vi "Select Active Channels.vi"(8 "error in (no error)":errorcluster, 9 "Impedance(s)":T1[](array[typedef]), 10 "Active Channel(s)":T2[](array[typedef]), 11 "MSOX6004 in":refnum<class "MSOX6004.lvclass">) -> (0 "error out":errorcluster, 3 "MSOX6004 out":refnum<class "MSOX6004.lvclass">)   [LabVIEW 2018, in "MSOX6004.lvlib" / "MSOX6004.lvclass"]
doc: "This Override method is used to set active channels for the Oscope. Use the 'Active Channel(s)' control to select channel(s)."
uses:
  MSOX6004.lvclass
  PPLs/Oscilloscope/Parent/Oscilloscope.lvlibp/Custom Controls/Analog Channels.ctl
  PPLs/Oscilloscope/Parent/Oscilloscope.lvlibp/Accessors/Channel Impedance.ctl
  MSOX6004.lvclass/MSOX6004.ctl
  <instrlib>/Keysight InfiniiVision/Keysight InfiniiVision.lvlib
  PPLs/Oscilloscope/Parent/Oscilloscope.lvlibp
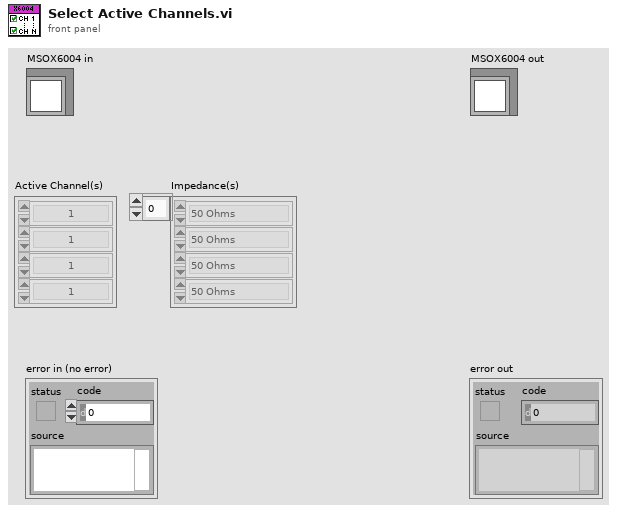
[diagram p1: front panel]
types:
  T1 = typedef "Oscilloscope.lvlibp/Channel Impedance.ctl" = enum16{"50 Ohms", "1 MOhms"}
  T2 = typedef "Oscilloscope.lvlibp/Analog Channels.ctl" = enum16{"1", "2", "3", "4", "5", "6", "7", "8", "9", "10", "11", "12", "13", "14", "15", "16"}
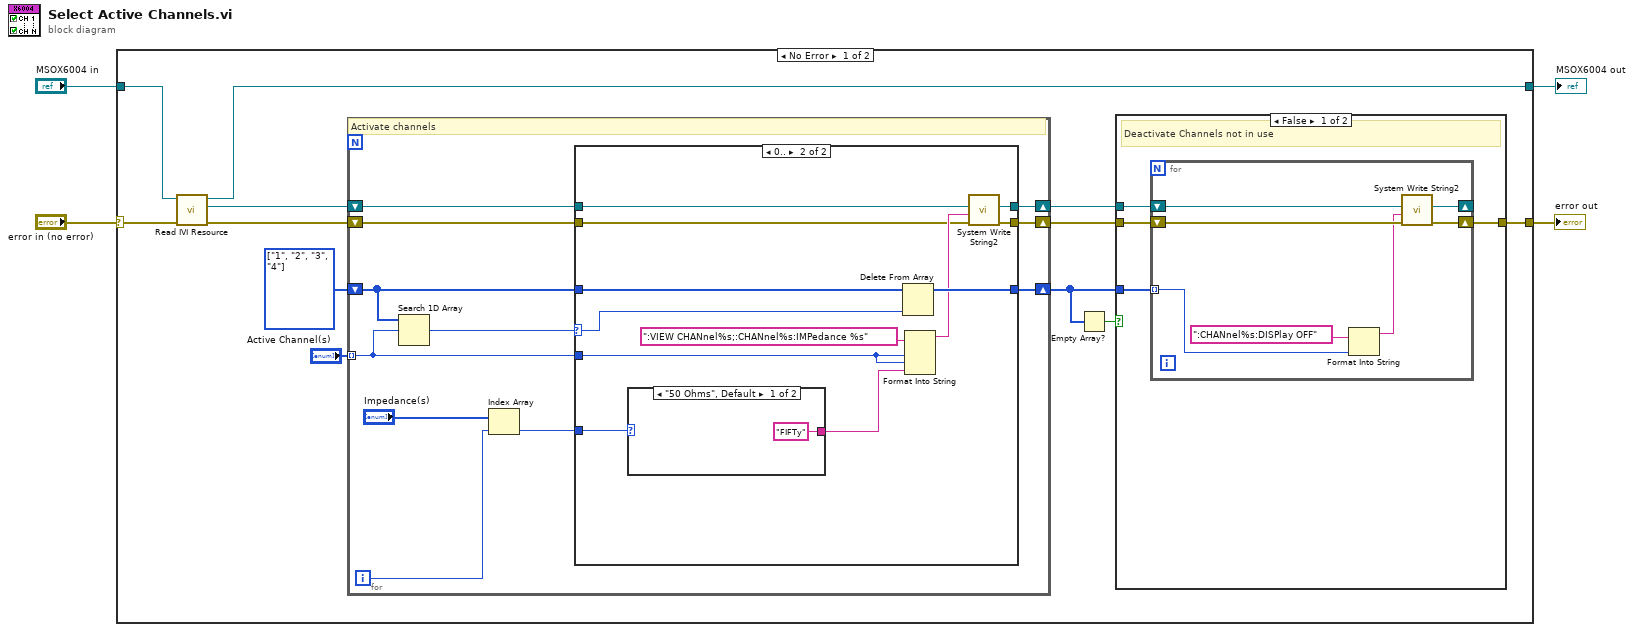
[diagram p0: block diagram]
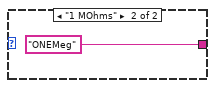
[diagram p4: hidden frame]
diagram:
  n1 = case shown="No Error" "error in (no error)" {
    selector: "error in (no error)" -> [w16 w57]
    tunnel: [w14 w58] -> w3
    tunnel: "MSOX6004 in" -> [w15 w58]
    tunnel: [w6 w57] -> w1
    frame No Error {
      w10 = T2[] [enum."1", enum."2", enum."3", enum."4"] items=["1", "2", "3", "4", "5", "6", "7", "8", "9", "10", "11", "12", "13", "14", "15", "16"] ("Active Channel(s)")
      n2 = call "Read IVI Resource.vi"("error in (no error)"=w16, "MSOX6004 in"=w15) -> ("error out"=w12:errorcluster, "IVI Resource"=w11:refnum<k15>, "MSOX6004 out"=w14:refnum<class "MSOX6004.lvclass">)  [unwired: 7 in]
      n3 = for {
        tunnel: "Active Channel(s)" -> [w38] mode=indexing
        shift-right: [w39] -> w7
        shift-left: w12 -> [w34]
        shift-right: [w35] -> w5
        shift-left: w10 -> [w36]
        shift-right: [w33] -> w8
        shift-left: w11 -> [w37]
        i -> [w29]
        # "Activate channels"
        n4 = Search 1D Array(1D array=w36, element=w38) -> (index of element=w31:i32)  [unwired: 1 in]
        n5 = Index Array(array="Impedance(s)", index=w29) -> (element=w30:T1)
        n6 = case shown="0.." w31 {
          selector: w31 -> [_ w50]
          tunnel: [w41 w54] -> w39
          tunnel: w38 -> [_ w44]
          tunnel: w37 -> [w42 w52]
          tunnel: w36 -> [w40 w51]
          tunnel: [w40 w49] -> w35
          tunnel: w34 -> [w41 w47]
          tunnel: [w42 w46] -> w33
          tunnel: w30 -> [_ w45]
          frame -1, Default {
          }
          frame 0.. {
            n7 = case shown="\"50 Ohms\", Default" w45 {
              tunnel: ["FIFTy" "ONEMeg"] -> w43
              frame "50 Ohms", Default {
              }
              frame "1 MOhms" {
              }
            }
            n8 = Delete From Array(array=w51, index=w50) -> (array with subset deleted=w49:T2[])  [unwired: 1 in, 1 out]
            n9 = Format Into String(format string=":VIEW CHANnel%s;:CHANnel%s:IMPedance %s", w44, w44, w43) -> (resulting string=w48:string)  [unwired: 2 in, 1 out]
            n10 = call <instrlib>:"System Write String2.vi"("error in (no error)"=w47, "Data"=w48, "instrument handle"=w52) -> ("error out"=w54:errorcluster, "instrument handle out"=w46:refnum<k15>)  [unwired: 7 in]
          }
        }
      }
      n11 = Empty Array?(array=w5) -> (empty?=w9:bool)
      n12 = case shown="False" w9 {
        tunnel: w8 -> [w19 _]
        tunnel: w7 -> [w18 w28]
        tunnel: [w17 w28] -> w6
        tunnel: w5 -> [w20 _]
        frame False {
          # "Deactivate Channels not in use"
          n13 = for {
            tunnel: w20 -> [w26] mode=indexing
            shift-right: [w24] -> _
            shift-left: w19 -> [w25]
            shift-right: [w22] -> w17
            shift-left: w18 -> [w23]
            n14 = Format Into String(format string=":CHANnel%s:DISPlay OFF", w26) -> (resulting string=w21:string)  [unwired: 2 in, 1 out]
            n15 = call <instrlib>:"System Write String2.vi"("error in (no error)"=w23, "Data"=w21, "instrument handle"=w25) -> ("error out"=w22:errorcluster, "instrument handle out"=w24:refnum<k15>)  [unwired: 7 in]
          }
        }
        frame True {
        }
      }
    }
    frame Error {
    }
  }
  "error out" <- w1
  "MSOX6004 out" <- w3
